vi "Delete_Fake_Dots_Array-3.vi"(2 "[IN] Dot matrix\nwith initial status":i16[][](array[numeric]), 3 "[IN] Source \nArray":dbl[][](array[numeric])) -> (0 "[OUT] Dot \nMatrix":i16[][](array[numeric]), 1 "[OUT] Filtered \nArray (X,Y)":dbl[][](array[numeric]))   [LabVIEW 2013]
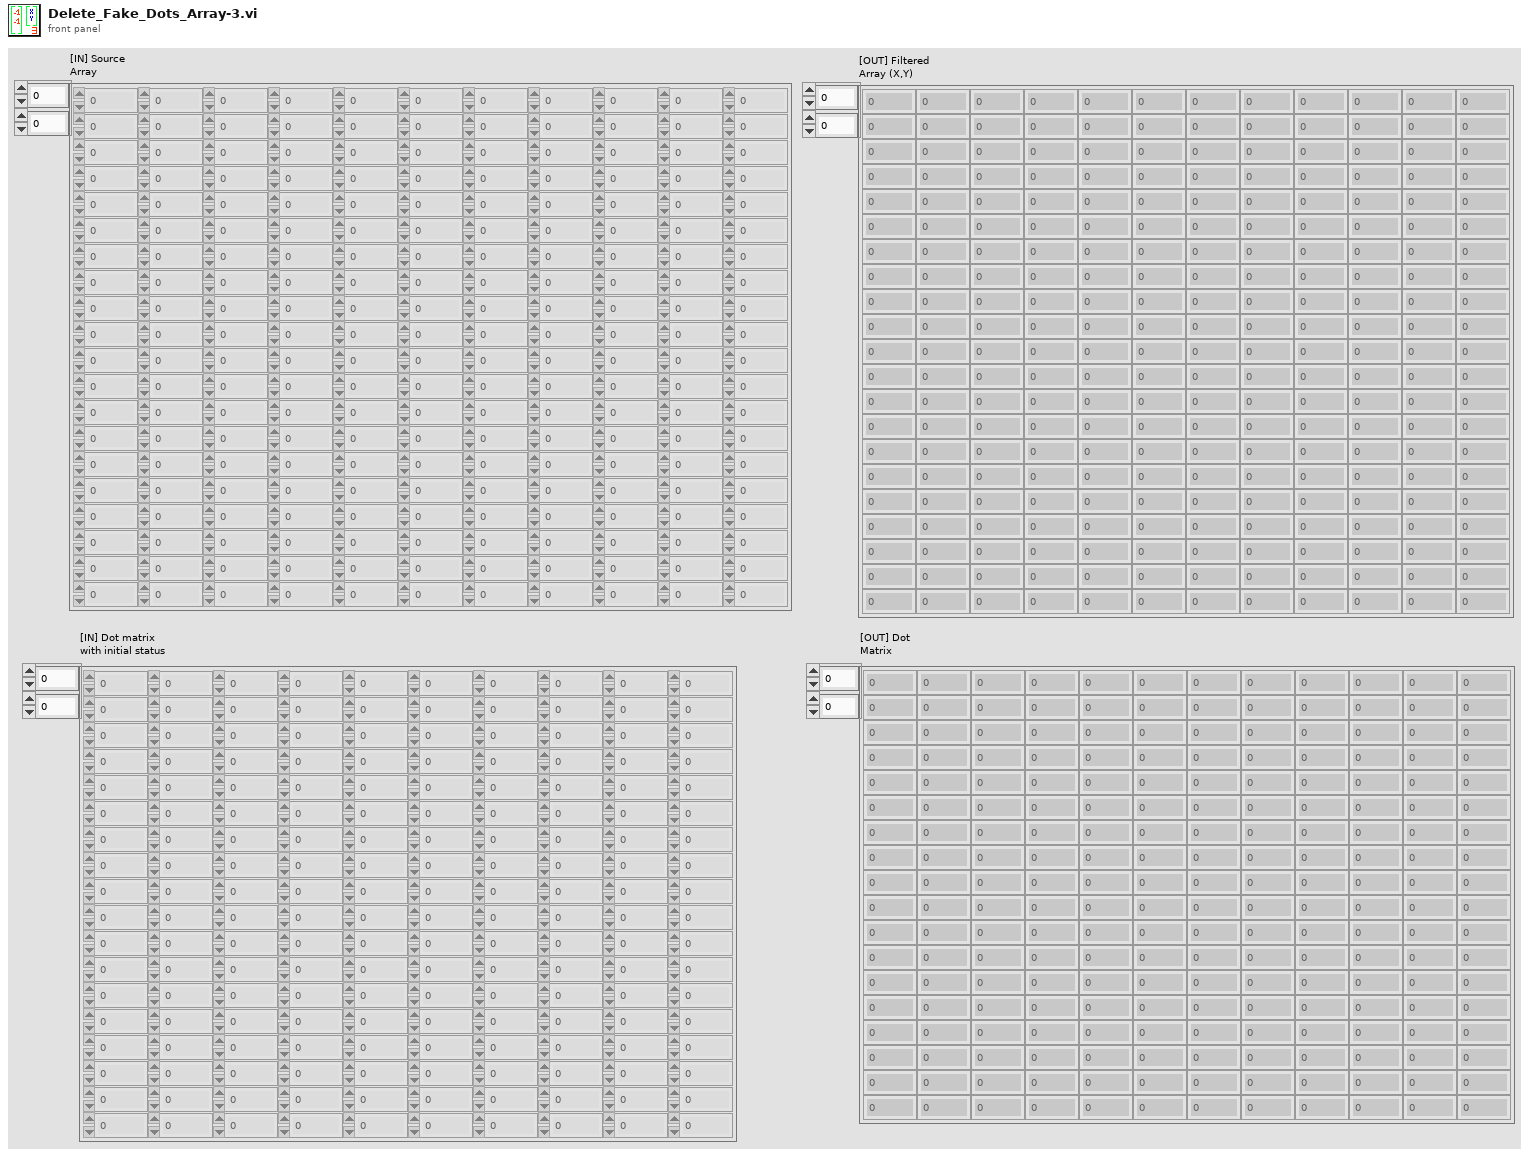
[diagram p1: front panel]
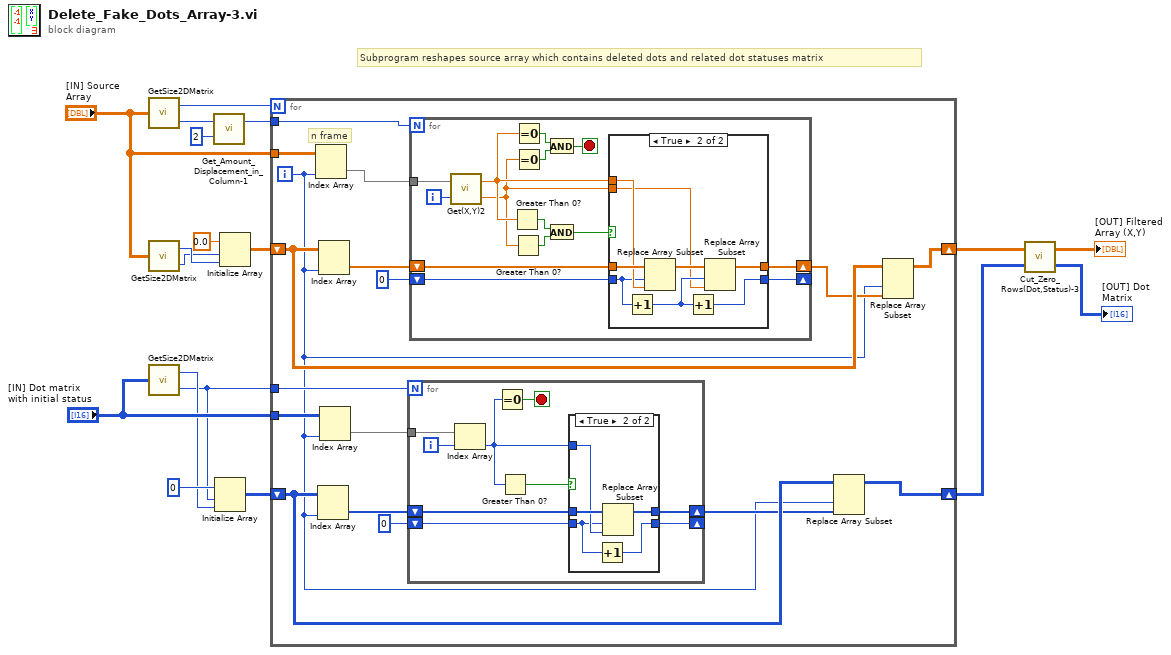
[diagram p0: block diagram]
diagram:
  # "Subprogram reshapes source array which contains deleted dots and related dot statuses matrix"
  n1 = call "GetSize2DMatrix.vi"("Array IN (2D)"="[IN] Source \nArray") -> ("# Cols"=w14:i32, "# Rows"=w12:i32)
  n2 = call "GetSize2DMatrix.vi"("Array IN (2D)"="[IN] Source \nArray") -> ("# Cols"=w17:i32, "# Rows"=w16:i32)
  n3 = call "GetSize2DMatrix.vi"("Array IN (2D)"="[IN] Dot matrix\nwith initial status") -> ("# Cols"=w7:i32, "# Rows"=w6:i32)
  n4 = call "Get_Amount_Displacement_in_Column-1.vi"("multiplier"=2 ("y"), "# Rows"=w12) -> ("Displ amount"=w10:i32)  [unwired: 1 out]
  n5 = Initialize Array(i16 0 ("element"), w6, w7) -> (w5:i16[][])
  n6 = Initialize Array(0.0 ("element"), w16, w17) -> (w15:dbl[][])
  n7 = for {
    N: w14 -> [_]
    tunnel: "[IN] Source \nArray" -> [w35]
    shift-right: [w31] -> w4
    shift-left: w15 -> [w32]
    tunnel: w10 -> [w28]
    tunnel: w6 -> [w25]
    shift-right: [w19] -> w2
    shift-left: w5 -> [w22]
    tunnel: "[IN] Dot matrix\nwith initial status" -> [w27]
    i -> [w20]
    # "n frame"
    n8 = Index Array(array=w35, index (col)=w20) -> (element=w33:dbl[])  [unwired: 1 in]
    n9 = Index Array(array=w22, index (col)=w20) -> (element=w24:i16[])  [unwired: 1 in]
    n10 = Index Array(array=w32, index (col)=w20) -> (element=w29:dbl[])  [unwired: 1 in]
    n11 = Index Array(array=w27, index (col)=w20) -> (element=w26:i16[])  [unwired: 1 in]
    n12 = for {
      N: w25 -> [_]
      tunnel: w26 -> [w44]
      shift-right: [w37] -> w21
      shift-left: w24 -> [w39]
      shift-right: [w36] -> _
      shift-left: 0 -> [w38]
      i -> [w43]
      stop <- w42 stop-if-true
      n13 = Index Array(array=w44, index=w43) -> (element=w40:i16)
      n14 = Equal To 0?(x=w40) -> (x = 0?=w42:bool)
      n15 = Greater Than 0?(x=w40) -> (x > 0?=w41:bool)
      n16 = case shown="True" w41 {
        tunnel: w40 -> [_ w50]
        tunnel: w39 -> [w46 w51]
        tunnel: w38 -> [w45 w48]
        tunnel: [w46 w49] -> w37
        tunnel: [w45 w47] -> w36
        frame False {
        }
        frame True {
          n17 = Increment(x=w48) -> (x+1=w47:i32)
          n18 = Replace Array Subset(array=w51, new element=w50, index=w48) -> (w49:i16[])
        }
      }
    }
    n19 = for {
      N: w28 -> [_]
      tunnel: w33 -> [w55]
      shift-right: [w56] -> w30
      shift-left: w29 -> [w59]
      shift-right: [w57] -> _
      shift-left: 0 -> [w58]
      i -> [w54]
      stop <- w63 stop-if-true
      n20 = call "Get(X,Y)2.vi"("[IN] index of (X,Y)"=w54, "[IN] Array coordi\nnates (X,Y) in Frame"=w55) -> ("[OUT] Y"=w52:dbl, "[OUT] X"=w53:dbl)
      n21 = Greater Than 0?(x=w53) -> (x > 0?=w62:bool)
      n22 = Greater Than 0?(x=w52) -> (x > 0?=w61:bool)
      n23 = Equal To 0?(x=w53) -> (x = 0?=w65:bool)
      n24 = Equal To 0?(x=w52) -> (x = 0?=w64:bool)
      n25 = And(x=w65, y=w64) -> (x .and. y?=w63:bool)
      n26 = And(x=w62, y=w61) -> (x .and. y?=w60:bool)
      n27 = case shown="True" w60 {
        tunnel: w59 -> [w67 w75]
        tunnel: w58 -> [w66 w73]
        tunnel: w53 -> [_ w74]
        tunnel: w52 -> [_ w70]
        tunnel: [w66 w68] -> w57
        tunnel: [w67 w69] -> w56
        frame False {
        }
        frame True {
          n28 = Increment(x=w73) -> (x+1=w71:i32)
          n29 = Replace Array Subset(array=w75, new element=w74, index=w73) -> (w72:dbl[])
          n30 = Increment(x=w71) -> (x+1=w68:i32)
          n31 = Replace Array Subset(array=w72, new element=w70, index=w71) -> (w69:dbl[])
        }
      }
    }
    n32 = Replace Array Subset(array=w22, new element=w21, index (col)=w20) -> (w19:i16[][])  [unwired: 1 in]
    n33 = Replace Array Subset(array=w32, new element=w30, index (col)=w20) -> (w31:dbl[][])  [unwired: 1 in]
  }
  n34 = call "Cut_Zero_Rows(Dot,Status)-3.vi"("[IN] Dot matrix\nwith zero points"=w2, "Array (X,Y) IN"=w4) -> ("[OUT] Dot \nMatrix"=→"[OUT] Dot \nMatrix":i16[][], "Array (X,Y) OUT"=→"[OUT] Filtered \nArray (X,Y)":dbl[][])
